vi "Histogram.vi"(7 "Last laser in":bool=TRUE, 9 "Histogram in":u16[](array[numeric])=[0, 0, 0, 0, 0, 0, 0, 0, 0, 0], 10 "PMT 60 in":bool[](array[boolean])=[FALSE, FALSE, FALSE, FALSE, FALSE, FALSE, FALSE, FALSE, FALSE, FALSE, FALSE, FALSE, FALSE, FALSE, FALSE, FALSE, FALSE, FALSE, FALSE, FALSE, FALSE, FALSE, FALSE, FALSE, FALSE, FALSE, FALSE, FALSE, FALSE, FALSE, FALSE, FALSE, FALSE, FALSE, FALSE, FALSE, FALSE, FALSE, FALSE, FALSE, FALSE, FALSE, FALSE, FALSE, FALSE, FALSE, FALSE, FALSE, FALSE, FALSE, FALSE, FALSE, FALSE, FALSE, FALSE, FALSE, FALSE, FALSE, FALSE, FALSE], 11 "Laser 60 in":bool[](array[boolean])=[FALSE, FALSE, FALSE, FALSE, FALSE, FALSE, FALSE, FALSE, FALSE, FALSE, FALSE, FALSE, FALSE, FALSE, FALSE, FALSE, FALSE, FALSE, FALSE, FALSE, FALSE, FALSE, FALSE, FALSE, FALSE, FALSE, FALSE, FALSE, FALSE, FALSE, FALSE, FALSE, FALSE, FALSE, FALSE, FALSE, FALSE, FALSE, FALSE, FALSE, FALSE, FALSE, FALSE, FALSE, FALSE, FALSE, FALSE, FALSE, FALSE, FALSE, FALSE, FALSE, FALSE, FALSE, FALSE, FALSE, FALSE, FALSE, FALSE, FALSE]) -> (1 "Histogram out":u16[](array[numeric]))   [LabVIEW 2012]
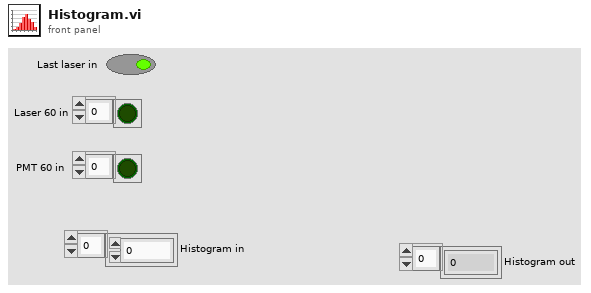
[diagram p1: front panel]
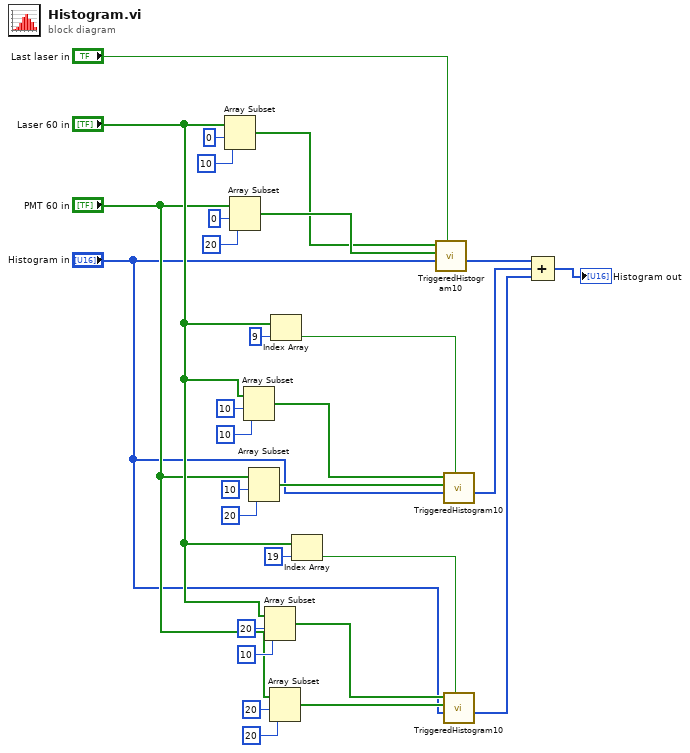
[diagram p0: block diagram]
diagram:
  n1 = Array Subset(array="Laser 60 in", index=0, length=10) -> (w24:bool[])
  n2 = Array Subset(array="PMT 60 in", index=0, length=20) -> (w25:bool[])
  n3 = Array Subset(array="Laser 60 in", index=10, length=10) -> (w18:bool[])
  n4 = Array Subset(array="PMT 60 in", index=10, length=20) -> (w19:bool[])
  n5 = Array Subset(array="Laser 60 in", index=20, length=10) -> (w7:bool[])
  n6 = Array Subset(array="PMT 60 in", index=20, length=20) -> (w8:bool[])
  n7 = Index Array(array="Laser 60 in", index=9) -> (element=w16:bool)
  n8 = Index Array(array="Laser 60 in", index=19) -> (element=w5:bool)
  n9 = call "TriggeredHistogram10.vi"("Last laser in"="Last laser in", "Histogram in"="Histogram in", "PMT 20bit in"=w25, "Laser 10bit in"=w24) -> ("Histogram out"=w15:u16[])  [unwired: 7 in]
  n10 = call "TriggeredHistogram10.vi"("Last laser in"=w16, "Histogram in"="Histogram in", "PMT 20bit in"=w19, "Laser 10bit in"=w18) -> ("Histogram out"=w14:u16[])  [unwired: 7 in]
  n11 = call "TriggeredHistogram10.vi"("Last laser in"=w5, "Histogram in"="Histogram in", "PMT 20bit in"=w8, "Laser 10bit in"=w7) -> ("Histogram out"=w4:u16[])  [unwired: 7 in]
  n12 = Compound Arithmetic op=ADD(w15, w14, w4) -> (→"Histogram out":u16[])
